vi "Write Duty Cycle.vi"(8 "error in (no error)":errorcluster, 10 "Duty Cycle (0‰)":u16, 11 "Heater in":refnum<class "Heater.lvclass">) -> (0 "error out":errorcluster, 3 "Heater out":refnum<class "Heater.lvclass">)   [LabVIEW 2015, in "cRIO-Carbondioxide.lvlib" / "CO2-Actor.lvlib" / "Heater.lvclass"]
uses:
  Heater.lvclass
  Heater.lvclass/Heater.ctl
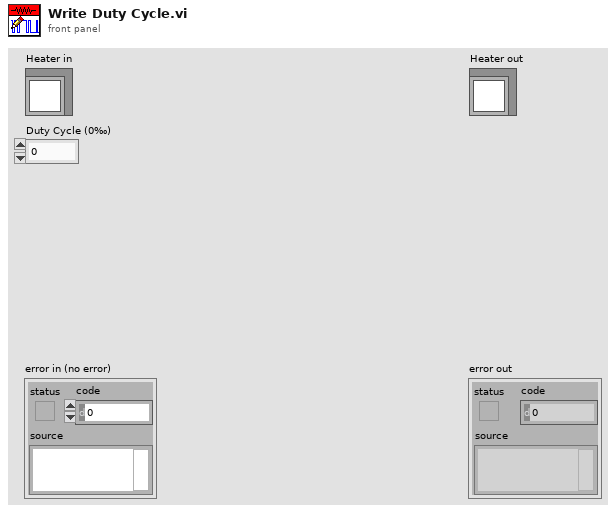
[diagram p1: front panel]
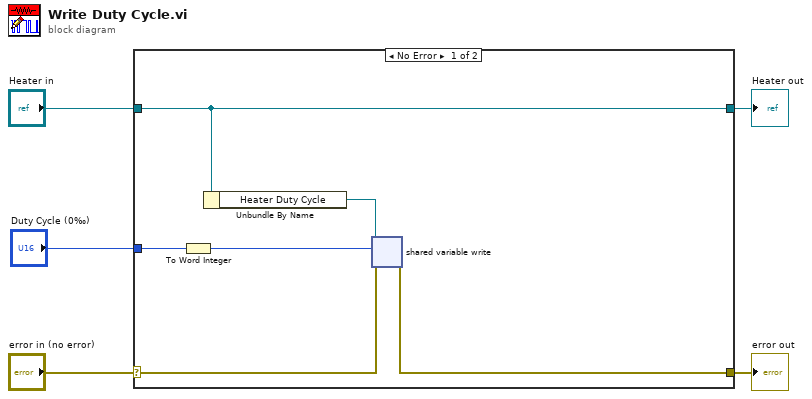
[diagram p0: block diagram]
diagram:
  n1 = case shown="No Error" "error in (no error)" {
    selector: "error in (no error)" -> [w7 w13]
    tunnel: [w6 w13] -> w4
    tunnel: [w11 w12] -> w2
    tunnel: "Heater in" -> [w11 w12]
    tunnel: "Duty Cycle (0‰)" -> [w9 _]
    frame No Error {
      n2 = To Word Integer(number=w9) -> (16bit integer=w8:i16)
      n3 = Unbundle By Name(w11) -> ("Heater Duty Cycle"=w10:refnum<k21>)
      n4 = shared-variable-write(w10, w7, w8) -> (w6:errorcluster)  [unwired: 1 out]
    }
    frame Error {
    }
  }
  "error out" <- w4
  "Heater out" <- w2
